vi "(Depricated) Open.vi"(6 "Interlock Chain":refnum<class "Interlock Chain.lvclass">=refnum, 8 "error in (no error)":errorcluster, 10 "index (All -1)":i32=-1, 11 "Valve in":refnum<class "Valve.lvclass">=refnum) -> (0 "error out":errorcluster, 3 "Valve out":refnum<class "Valve.lvclass">)   [LabVIEW 2015]
uses:
  Valve.lvclass
  Interlocks/Interlock Chain/Interlock Chain.lvclass
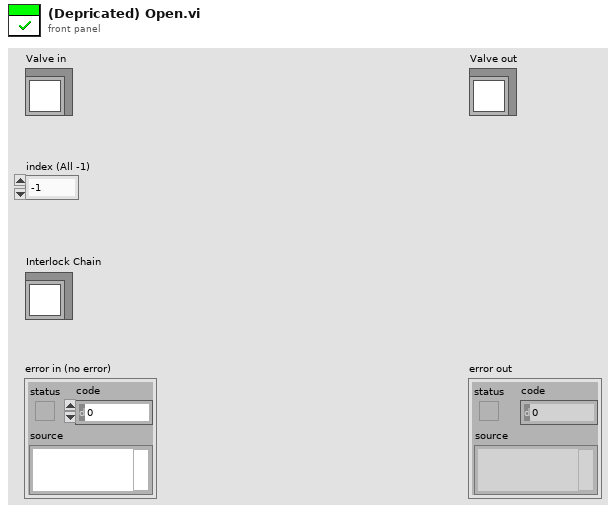
[diagram p1: front panel]
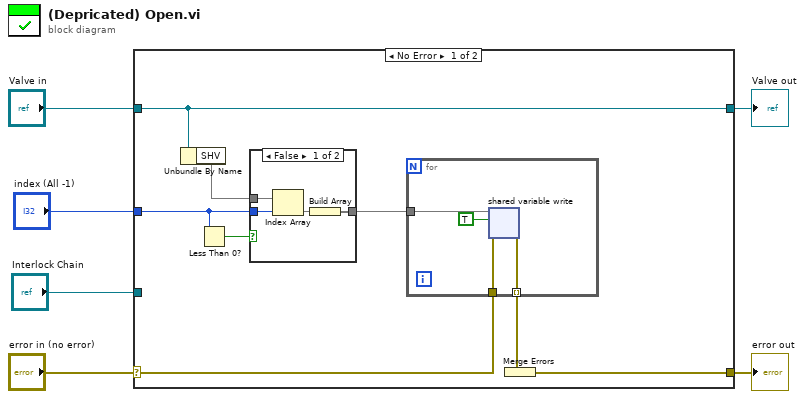
[diagram p0: block diagram]
diagram:
  n1 = case shown="No Error" "error in (no error)" {
    selector: "error in (no error)" -> [w13 w25]
    tunnel: [w7 w25] -> w5
    tunnel: [w14 w24] -> w3
    tunnel: "Valve in" -> [w14 w24]
    tunnel: "Interlock Chain" -> [_ _]
    tunnel: "index (All -1)" -> [w9 _]
    frame No Error {
      n2 = Unbundle By Name(w14) -> ("SHV"=w10)
      n3 = Less Than 0?(x=w9) -> (x < 0?=w8:bool)
      n4 = case shown="False" w8 {
        tunnel: [w19 w23] -> w11
        tunnel: w9 -> [w21 _]
        tunnel: w10 -> [w20 w23]
        frame False {
          n5 = Index Array(array=w20, index=w21) -> (element=w22)
          n6 = Build Array(w22) -> (w19:void[])
        }
        frame True {
        }
      }
      n7 = for {
        tunnel: w13 -> [w17]
        tunnel: [w16] -> w12 mode=indexing
        tunnel: w11 -> [w15]
        n8 = shared-variable-write(w15, w17, TRUE) -> (w16:errorcluster)  [unwired: 1 out]
      }
      n9 = Merge Errors(w12) -> (w7:errorcluster)
    }
    frame Error {
    }
  }
  "error out" <- w5
  "Valve out" <- w3
